vi "Global Refnums.vi"() -> ()   [LabVIEW 2012]
panel:
  out "Jaw":string
  out "Mid Foot":string
  out "Back Leg PS":string
  out "Arm":string
  out "Mid Leg PS":string
  out "Front Leg PS":string
  out "Front Foot":string
  out "Back Claw":string
  out "Mid Claw":string
  out "Front Claw":string
  out "Skids":string
  out "Back Leg Up":string
  out "Front Leg Up":string
  out "Mid Leg Up":string
  out "Climb/ Shoot":string
  out "Shooter Elevation":string
  out "Shooter Pusher":string
  out "Cheat Code":string
  out "Compressor":string
  out "Joystick R 2":string
  out "Joystick L 1":string
  out "Rotational Motor BL":string
  out "Rotational Motor BR":string
  out "Rotational Motor FL":string
  out "Rotational Motor FR":string
  out "Drive Motor BL":string
  out "Drive Motor BR":string
  out "Drive Motor FL":string
  out "Drive Motor FR":string
  out "V Encoder BL":string
  out "V Encoder BR":string
  out "V Encoder FL":string
  out "V Encoder FR":string
  out "A Encoder BL":string
  out "A Encoder BR":string
  out "A Encoder FL":string
  out "A Encoder FR":string
  # "Caterpillar"
  # "Encoders"
  # "Motors"
  # "Joysticks"
  # "Cheat Code"
  # "Climb/ Shoot"
  # "Arm"
  # "(Really caterpillar motor)"
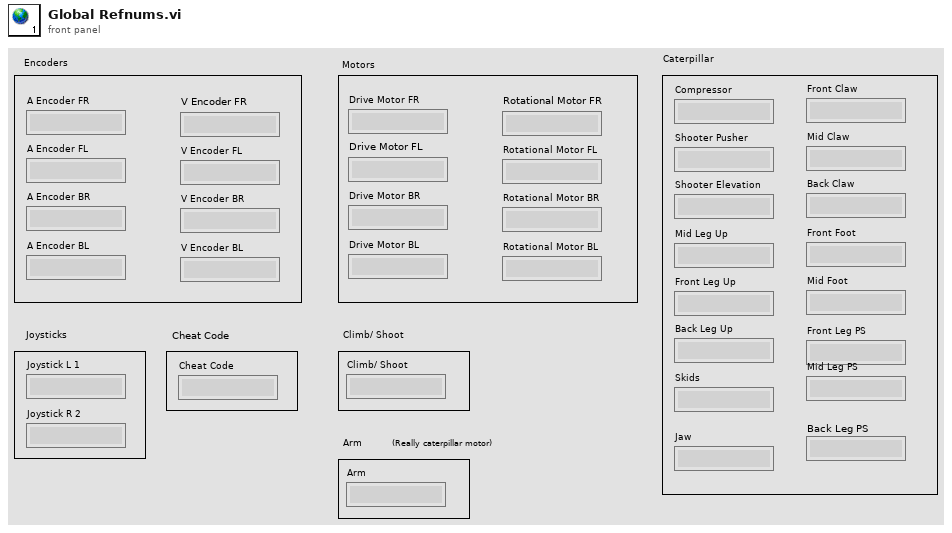
[diagram p1: front panel]
diagram:
